vi "Range1.vi"() -> ()   [LabVIEW 2019]
uses:
  Supported.llb/Global-1.vi
panel:
  out "Slide":cluster{dbl, dbl}(slide) scale=-10.0..10.0
  out "Upper":dbl
  out "Lower":dbl
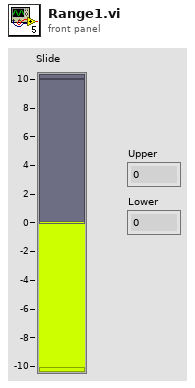
[diagram p1: front panel]
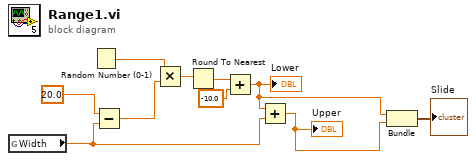
[diagram p0: block diagram]
diagram:
  n1 = global read "Global-1.vi" "Width"() -> (w1:dbl)
  n2 = Random Number (0-1)() -> (number: 0 to 1=w10:dbl)
  n3 = Subtract(x=20.0, y=w1) -> (x-y=w2:dbl)
  n4 = Multiply(x=w10, y=w2) -> (x*y=w9:dbl)
  n5 = Round To Nearest(number=w9) -> (nearest integer value=w8:dbl)
  n6 = Add(x=w8, y=-10.0) -> (x+y=w6:dbl)
  "Lower" <- w6
  n7 = Add(x=w6, y=w1) -> (x+y=w5:dbl)
  "Upper" <- w5
  n8 = Bundle(w6, w5) -> (→"Slide":cluster{dbl, dbl})  [unwired: 1 in]
